vi "Module Cleanup.vi"(8 "error in (no error)":errorcluster, 11 "GenericGuiDI in":refnum<class "GenericGuiDI.lvclass">) -> (0 "error out":errorcluster, 3 "GenericGuiDI out":refnum<class "GenericGuiDI.lvclass">)   [LabVIEW 2020, in "VolatusDAQGenericGUI.lvlib" / "GenericGuiDI.lvclass"]
uses:
  GenericGuiDI.lvclass
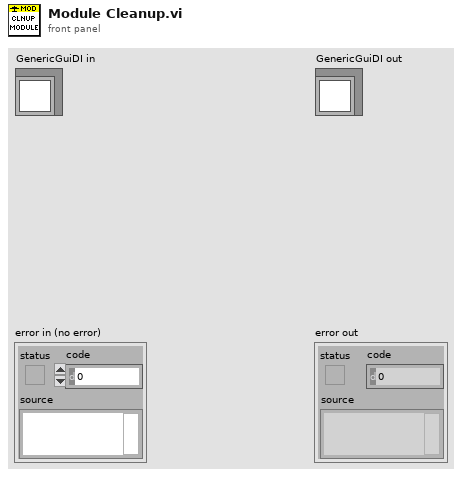
[diagram p1: front panel]
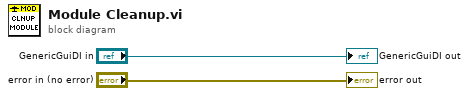
[diagram p0: block diagram]
diagram:
  "error out" <- "error in (no error)"
  "GenericGuiDI out" <- "GenericGuiDI in"
